vi "Read Date from SnP File.vi"(0 "Result File Path":path, 11 "error in (no error)":errorcluster) -> (4 "Result File Path Out":path, 6 "Path Charact Date":timestamp, 15 "error out":errorcluster)   [LabVIEW 2023, in "RFFixtureCharact.RFPM.lvlib" / "Charact Result Accessor.lvclass"]
uses:
  Charact Result Accessor.lvclass
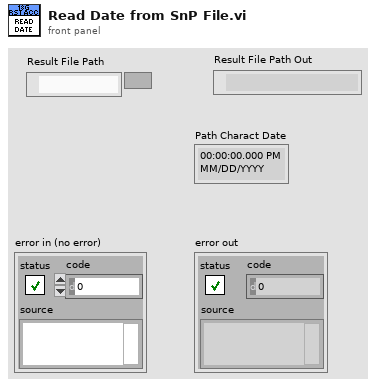
[diagram p1: front panel]
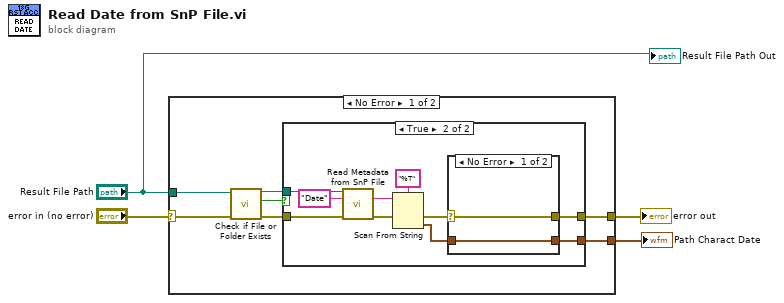
[diagram p0: block diagram]
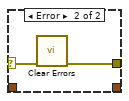
[diagram p3: hidden frame]
diagram:
  n1 = case shown="No Error" "error in (no error)" {
    selector: "error in (no error)" -> [w6 w27]
    tunnel: [w11 w27] -> w3
    tunnel: [w7 _] -> w2
    tunnel: "Result File Path" -> [w5 _]
    frame No Error {
      n2 = call <vilib>:"Check if File or Folder Exists.vi"("error in (no error)"=w6, "path"=w5) -> ("error out"=w10:errorcluster, "file or folder exists?"=w8:bool, "dup path"=w9:path)  [unwired: 7 in]
      n3 = case shown="True" w8 {
        tunnel: [w12 w13] -> w11
        tunnel: w10 -> [w12 w18]
        tunnel: w9 -> [_ w17]
        tunnel: [_ w15] -> w7
        frame False {
        }
        frame True {
          n4 = call "Read Metadata from SnP File.vi"("SnP File Path in"=w17, "Key"="Date", "error in (no error)"=w18) -> ("Value"=w20:string, "error out"=w21:errorcluster)  [unwired: 10 in, 1 out]
          n5 = Scan From String(format string="%T", input string=w20, error in=w21) -> (error out=w16:errorcluster, output 1=w14:timestamp)  [unwired: 2 in, 2 out]
          n6 = case shown="No Error" w16 {
            selector: w16 -> [w23 w26]
            tunnel: [w24 _] -> w15
            tunnel: w14 -> [w24 _]
            tunnel: [w23 w25] -> w13
            frame No Error {
            }
            frame Error {
              n7 = call <vilib>:"Clear Errors.vi"("error in (no error)"=w26) -> ("error out"=w25:errorcluster)  [unwired: 5 in, 1 out]
            }
          }
        }
      }
    }
    frame Error {
    }
  }
  "error out" <- w3
  "Path Charact Date" <- w2
  "Result File Path Out" <- "Result File Path"
